vi "找一字槽方向-两头缺口.vi"(9 "Fitted Circle":T1, 11 "Img in":T2) -> (1 "一字槽角度":dbl, 3 "一字槽中心":cluster{"X":sgl, "Y":sgl}, 4 "半径+槽宽+角度差异mm":dbl[](array[numeric]))   [LabVIEW 2014]
uses:
  <vilib>/vision/Measure.llb/Edge Options.ctl
  <vilib>/vision/Measure.llb/Edge Polarity.ctl
  <vilib>/vision/Image Controls.llb/IMAQ Image.ctl
  Global.vi
panel:
  out "角度差异数组(任意一个满足即可)":dbl[](array[numeric])
  in  "画搜索线?":bool
  out "一字槽宽度":dbl
  out "存储缺口中心位置":cluster{"X":sgl, "Y":sgl}[](array[cluster])
  out "圆心到边距离 2":sgl[][](graph)
  out "缺口数量":i32
  in  "Options":T3={"Edge Polarity"=2, "Kernel Size"=7, "Width"=7, "Minimum Edge Strength"=20.0, "Interpolation Type"=enum."Bilinear Fixed", "Data Processing Method"=enum."Average"} {"Edge Polarity" items=["All Edges", "Rising Edges", "Falling Edges"]; "Minimum Edge Strength" format="%.2f"; "Width" step=2; "Kernel Size" step=2}
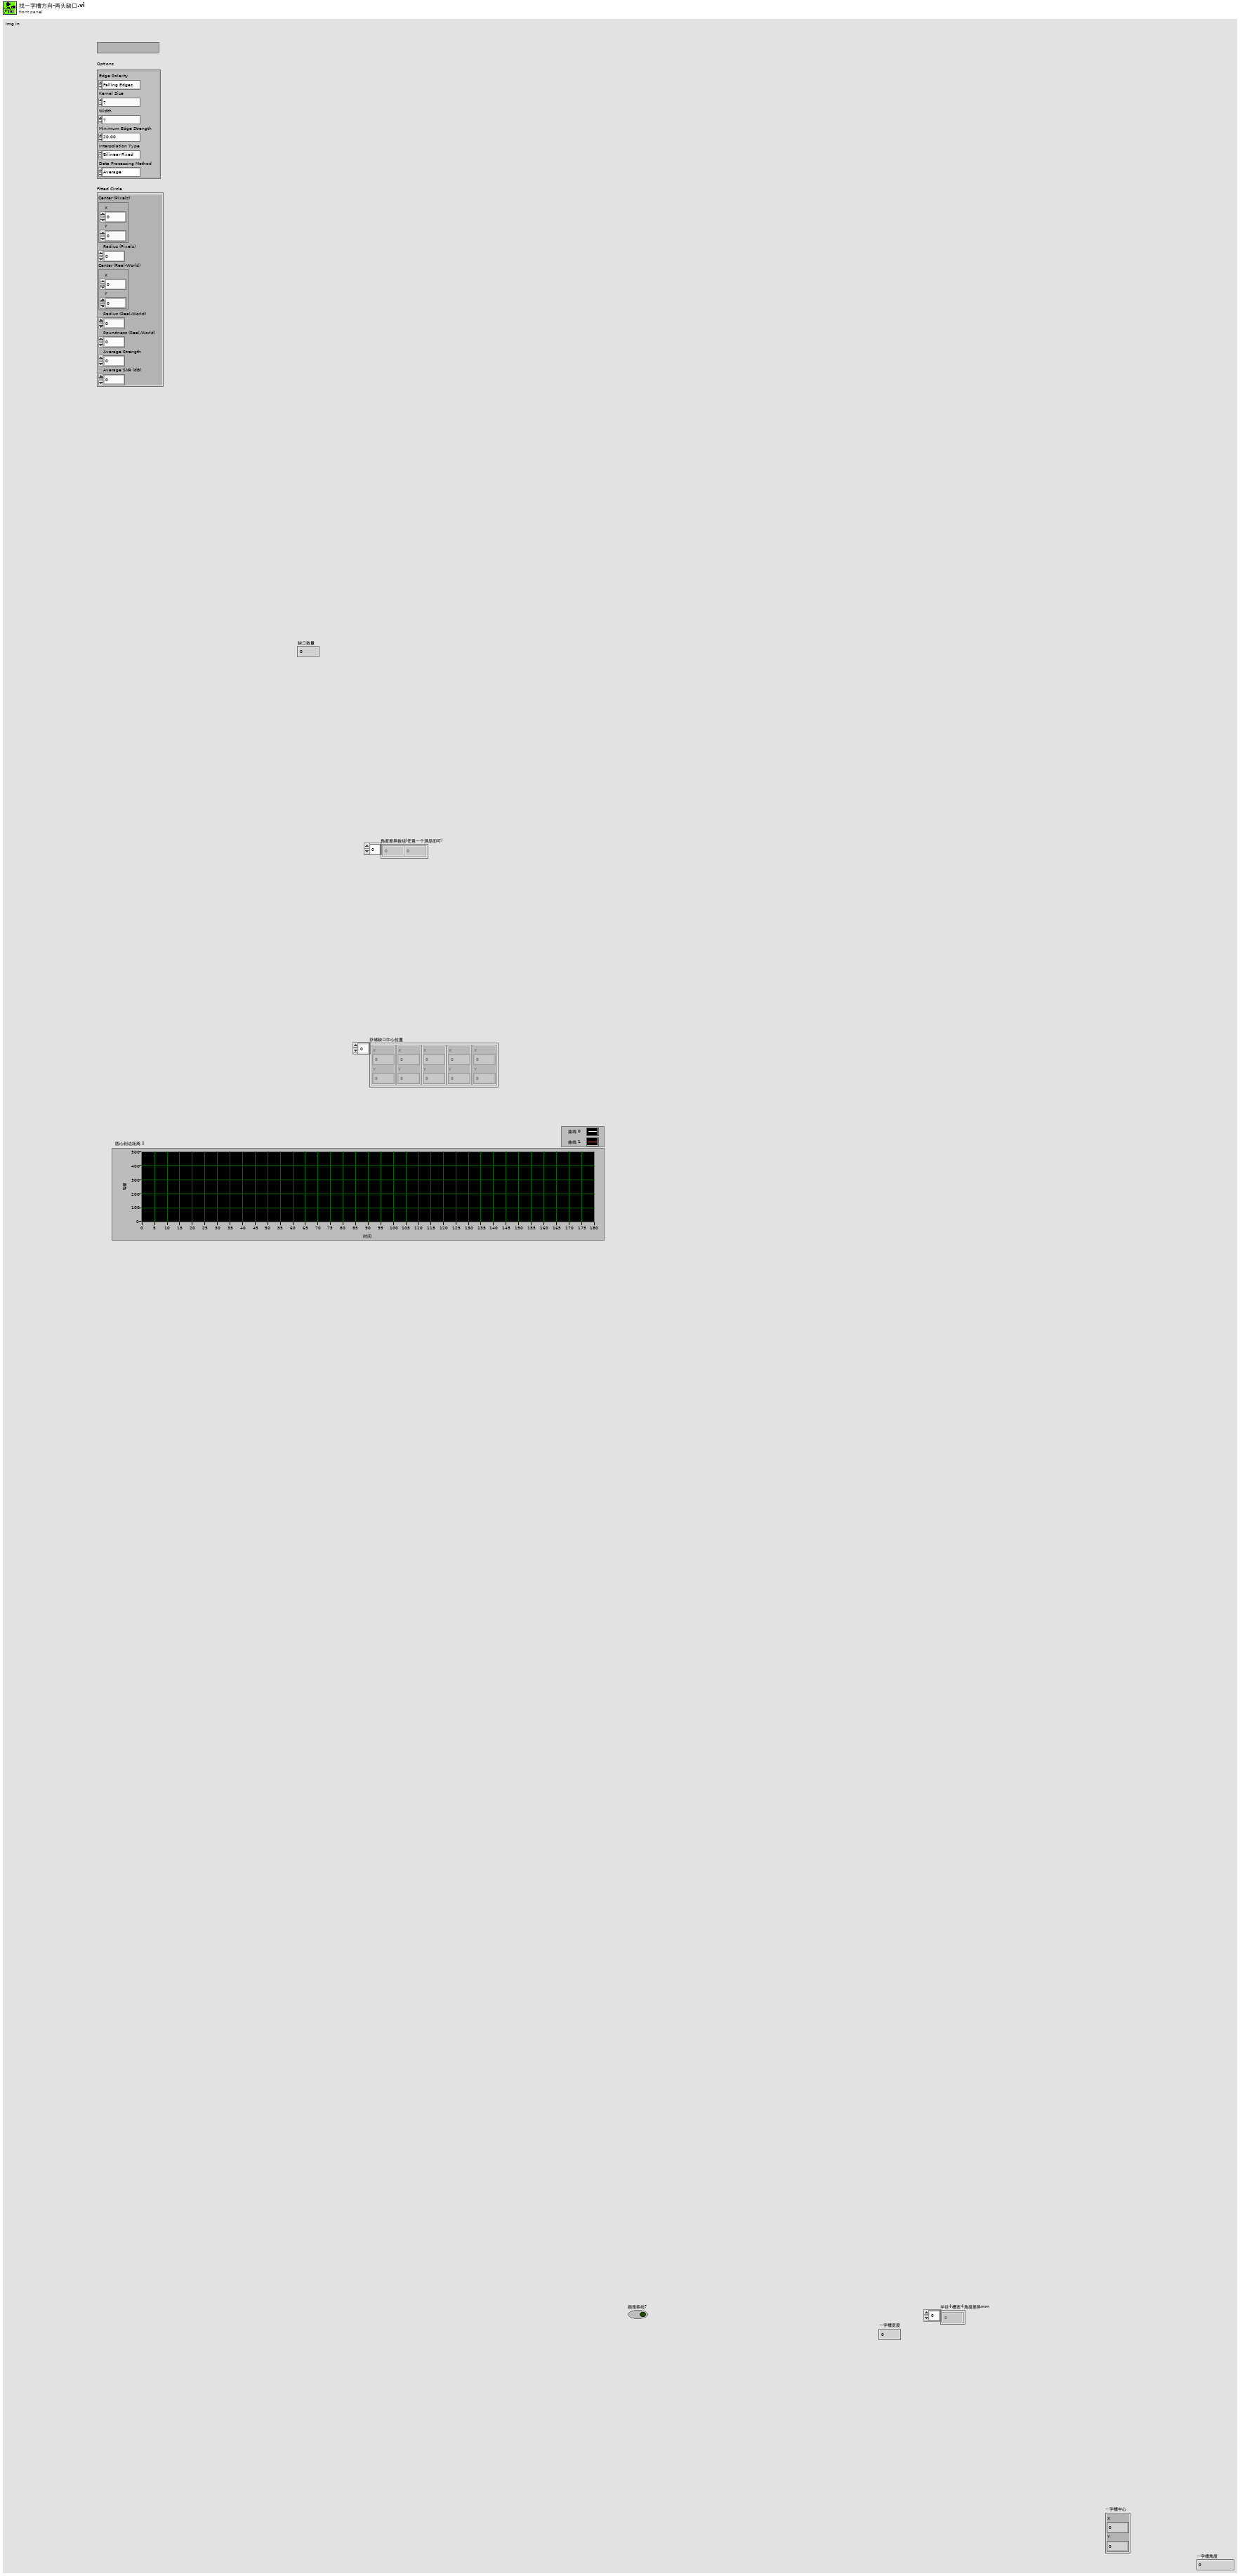
[diagram p1: front panel]
types:
  T1 = cluster{"Center (Pixels)":cluster{"X":sgl, "Y":sgl}, "Radius (Pixels)":dbl, "Center (Real-World)":cluster{"X":sgl, "Y":sgl}, "Radius (Real-World)":dbl, "Roundness (Real-World)":dbl, "Average Strength":dbl, "Average SNR (dB)":dbl}
  T2 = typedef "IMAQ Image.ctl" = refnum<image>
  T3 = typedef "Edge Options.ctl" = cluster{"Edge Polarity":T4, "Kernel Size":u32, "Width":u32, "Minimum Edge Strength":sgl, "Interpolation Type":enum32{"Zero Order", "Bilinear", "Quadratic", "Cubic", "Bilinear Fixed"}, "Data Processing Method":enum32{"Average", "Median"}}
  T4 = typedef "Edge Polarity.ctl" = u32
  T5 = typedef "ROI Descriptor" = cluster{"Global Rectangle":i32[], "Contours":cluster{"ID":enum32{"External", "Internal"}, "Type":u32, "Coordinates":i32[]}[]}
  T6 = typedef "OtherSpec.ctl" = cluster{"其它勾选类规格":T7, "其它数据类规格":T8, "相机名称":T9, "参数":cluster{"Mark1曝光时间":i32, "Mark2曝光时间":i32, "二维码曝光时间":i32}}
  T7 = typedef "其它勾选类规格.ctl" = cluster{"保存图片":bool, "上传设备状态数据":bool, "保存数据":bool, "开机默认开启监控摄像头":bool, "启用mark拍照 ":bool}
  T8 = typedef "其他数据类规格.ctl" = cluster{"相机1像素-毫米换算系数":dbl, "相机2像素-毫米换算系数":dbl, "D盘剩余空间预警(G)":dbl, "视频最长录制时间(秒)":dbl}
  T9 = typedef "相机名称品牌使用状态.ctl" = cluster{"相机1名称":T10, "相机2名称":T10, "Cam1启用":bool, "Cam2启用":bool, "Basler1":bool, "Basler2":bool}
  T10 = typedef "IMAQdx.ctl" = refnum<k21>
  T11 = cluster{"Point 1":cluster{"X":sgl, "Y":sgl}, "Point 2":cluster{"X":sgl, "Y":sgl}}
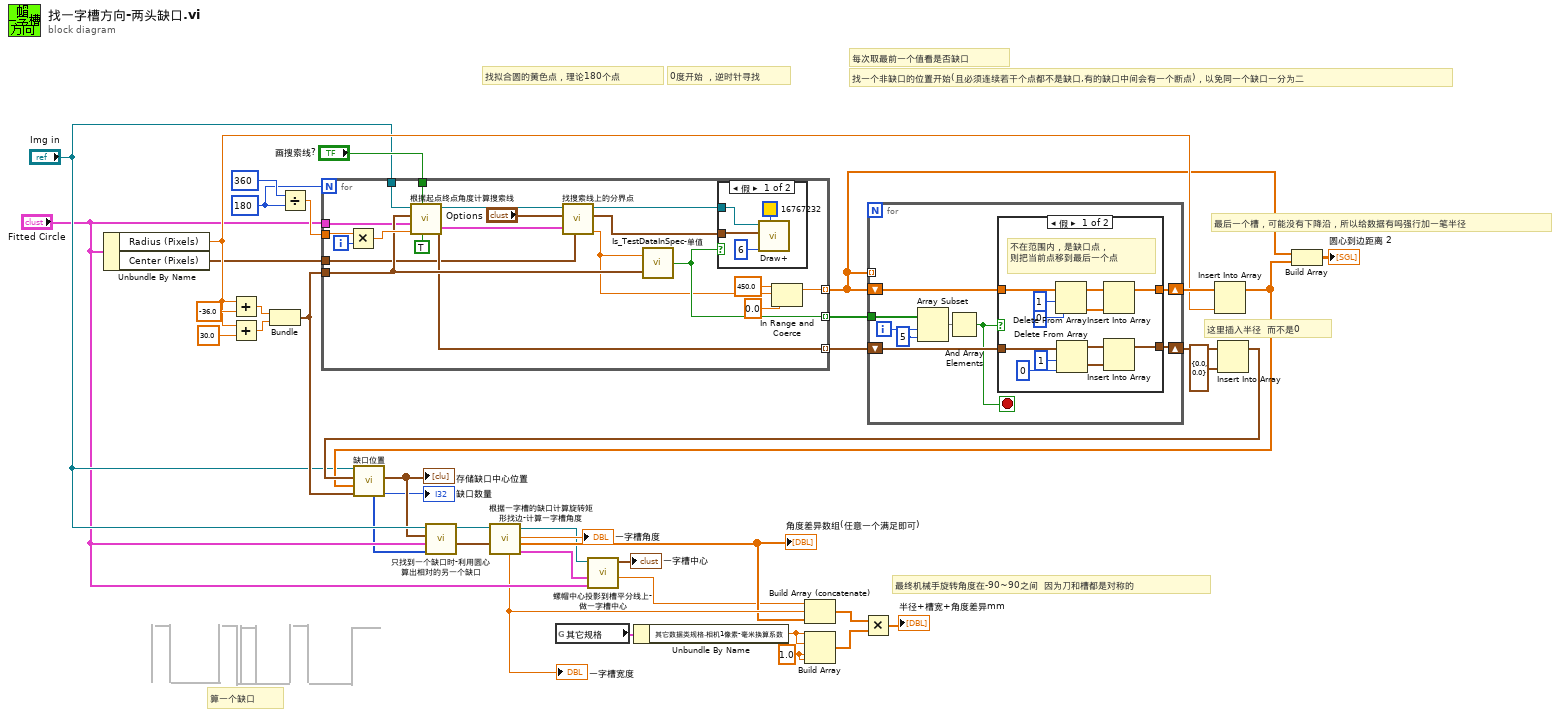
[diagram p0: block diagram]
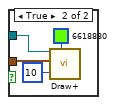
[diagram p3: hidden frame]
diagram:
  w1 = 1.0 ("元素")
  w29 = 180
  # "最终机械手旋转角度在-90~90之间  因为刀和槽都是对称的"
  # "算一个缺口"
  # "0度开始 ，逆时针寻找"
  # "这里插入半径  而不是0"
  # "最后一个槽，可能没有下降沿，所以给数据有吗强行加一笔半径"
  # "每次取最前一个值看是否缺口"
  # "找拟合圆的黄色点，理论180个点"
  # "找一个非缺口的位置开始(且必须连续若干个点都不是缺口,有的缺口中间会有一个断点)，以免同一个缺口一分为二"
  n1 = Unbundle By Name("Fitted Circle") -> ("Radius (Pixels)"=w28:dbl, "Center (Pixels)"=w21:cluster{"X":sgl, "Y":sgl})
  n2 = Add(x=w28, y=-36.0) -> (x+y=w25:dbl)
  n3 = Add(x=w28, y=30.0) -> (x+y=w24:dbl)
  n4 = Bundle(w25, w24) -> (w23:cluster{dbl, dbl})  [unwired: 1 in]
  n5 = Divide(x=360, y=w29) -> (x/y=w40:dbl)
  n6 = for "For循环" {
    N: w29 -> [_]
    tunnel: "Fitted Circle" -> [w48]
    tunnel: "Img in" -> [w46]
    tunnel: w40 -> [w59]
    tunnel: [w55] -> w26 mode=indexing
    tunnel: [w49] -> w38 mode=indexing
    tunnel: [w50] -> w27 mode=indexing
    tunnel: w23 -> [w51]
    tunnel: "画搜索线?" -> [w47]
    tunnel: w21 -> [w42]
    i -> [w60]
    n7 = Multiply(x=w59, y=w60) -> (x*y=w54:dbl)
    n8 = call "根据起点终点角度计算搜索线.vi"("从内外外搜索"=TRUE, "画搜索线?"=w47, "角度"=w54, "Fitted Circle"=w48, "内径外径"=w51, "Img in"=w46) -> ("ROI 找边"=w52:T5, "找不到边界时默认点"=w49:cluster{dbl, dbl}, "Img out"=w44:T2)  [unwired: 3 in]
    n9 = call "找搜索线上的分界点.vi"("圆心"=w42, "ROI 找边"=w52, "Options"="Options", "引用句柄输入"=w44) -> ("两点之间距离"=w41:sgl, "Location (Pixel)"=w43:cluster{"X":sgl, "Y":sgl}, "引用句柄输出"=w45:T2)  [unwired: 5 in]
    n10 = call "Is_TestDataInSpec-单值.vi"("量测规格"=w51, "相机量测结果"=w41) -> ("在规格内"=w50:bool)
    n11 = case shown="假" w50 {
      tunnel: w45 -> [w63 w68]
      tunnel: w43 -> [w62 w67]
      frame False {
        n12 = call "Draw+.vi"("Width"=6, "Color"=u32 16767232, "input cluster"=w62, "Image In"=w63) -> ()  [unwired: 2 in, 1 out]
      }
      frame True {
        n13 = call "Draw+.vi"("Width"=10, "Color"=u32 6618880, "input cluster"=w67, "Image In"=w68) -> ()  [unwired: 2 in, 1 out]
      }
    }
    n14 = In Range and Coerce(upper limit=sgl 450.0 ("上限"), x=w41, lower limit=sgl 0.0 ("下限")) -> (coerced(x)=w55:sgl)  [unwired: 1 out]
  }
  n15 = global read "Global.vi" "其它规格"() -> (w7:T6)
  n16 = Unbundle By Name(w7) -> ("其它数据类规格.相机1像素-毫米换算系数"=w6:dbl)
  n17 = Build Array(w6, w6, w1, w1) -> (w4:dbl[])
  n18 = for {
    tunnel: w26 -> [_] mode=indexing
    shift-right: [w77] -> w35
    shift-left: w38 -> [w75]
    shift-right: [w76] -> w36
    shift-left: w26 -> [w74]
    tunnel: w27 -> [w73]
    i -> [w71]
    stop <- w69 stop-if-true
    n19 = Array Subset(array=w73, index=w71, length=5 ("索引")) -> (w70:bool[])
    n20 = And Array Elements(Boolean array=w70) -> (logical AND=w69:bool)
    n21 = case shown="假" w69 {
      tunnel: w75 -> [w89 w90]
      tunnel: [w88 w90] -> w77
      tunnel: w74 -> [w85 w91]
      tunnel: [w84 w91] -> w76
      frame False {
        # "不在范围内，是缺口点，\n则把当前点移到最后一个点"
        n22 = Delete From Array(array=w85, length=1 ("长度"), index=0 ("索引")) -> (deleted portion=w78:sgl[], array with subset deleted=w87:sgl[])
        n23 = Delete From Array(array=w89, length=1 ("长度"), index=0 ("索引")) -> (deleted portion=w79:cluster{dbl, dbl}[], array with subset deleted=w82:cluster{dbl, dbl}[])
        n24 = Insert Into Array ("数组插入")(array=w87, new element=w78) -> (w84:sgl[])  [unwired: 1 in]
        n25 = Insert Into Array ("数组插入")(array=w82, new element=w79) -> (w88:cluster{dbl, dbl}[])  [unwired: 1 in]
      }
      frame True {
      }
    }
  }
  n26 = Insert Into Array(array=w36, new element=w28) -> (w33:sgl[])  [unwired: 1 in]
  n27 = Insert Into Array(array=w35, new element=cluster{dbl, dbl} {0.0, 0.0} ("新元素/子数组")) -> (w34:cluster{dbl, dbl}[])  [unwired: 1 in]
  n28 = call "缺口位置.vi"("是否缺口判断标准"=w23, "圆心到分界点半径"=w33, "分界点坐标"=w34, "Img输入"="Img in") -> ("缺口数量"=→"缺口数量":i32, "存储缺口中心位置"=w19:cluster{"X":sgl, "Y":sgl}[], "每个缺口像素点数量"=w14:i32[])  [unwired: 5 in]
  "存储缺口中心位置" <- w19
  n29 = call "只找到一个缺口时-利用圆心算出相对的另一个缺口.vi"("每个缺口像素点数量"=w14, "Fitted Circle"="Fitted Circle", "存储缺口位置in"=w19, "img in"="Img in") -> ("存储缺口位置 out"=w17:cluster{"X":sgl, "Y":sgl}[], "img out"=w18:T2)  [unwired: 6 in]
  n30 = call "根据一字槽的缺口计算旋转矩形找边-计算一字槽角度.vi"("存储缺口位置 out"=w17, "Img输入"=w18) -> ("一字槽角度线"=w10:T11, "角度差异"=w11:dbl[], "一字槽角度"=→"一字槽角度":dbl, "Img out"=w9:T2, "一字槽宽度"=w12:dbl)  [unwired: 5 in]
  "一字槽宽度" <- w12
  "角度差异数组(任意一个满足即可)" <- w11
  n31 = call "螺帽中心投影到槽平分线上-做一字槽中心.vi"("Fitted Circle"="Fitted Circle", "一字槽两边的角平分线"=w10, "Image In"=w9) -> ("Radius (Pixels)"=w8:dbl, "一字槽中心"=→"一字槽中心":cluster{"X":sgl, "Y":sgl})  [unwired: 7 in]
  n32 = Build Array (concatenate)(w8, w12, w11) -> (w5:dbl[])
  n33 = Multiply(x=w5, y=w4) -> (x*y=→"半径+槽宽+角度差异mm":dbl[])
  n34 = Build Array(w26, w33) -> (→"圆心到边距离 2":sgl[][])
